vi "shooter_open.vi"(8 "error in (no error)":errorcluster) -> (0 "error out":errorcluster)   [LabVIEW 2020]
uses:
  <vilib>/Rock Robotics/WPI/ThirdParty/Phoenix-LabVIEW/Motor Controller/Controls/CTRE_Phoenix_MotorControl_NeutralMode.ctl
  Robot Global Data.vi
  <vilib>/Rock Robotics/WPI/ThirdParty/REV Robotics/REVLib/Typedef/Spark MAX Idle Mode.ctl
panel:
  in  "Turret PIDF Constants":T1={"Set Constants"=TRUE, "P"=0.02, "I"=0.0001, "D"=0.0, "F"=0.0, "I Zone"=0.0, "Cruise Velocity"=50000, "Acceleration"=50000, "Percent Deadband"=0.0}
  in  "Flywheel PIDF Constants":T1={"Set Constants"=TRUE, "P"=0.00029748, "I"=0.0, "D"=0.0, "F"=0.0, "I Zone"=0.0, "Cruise Velocity"=0, "Acceleration"=0, "Percent Deadband"=0.0}
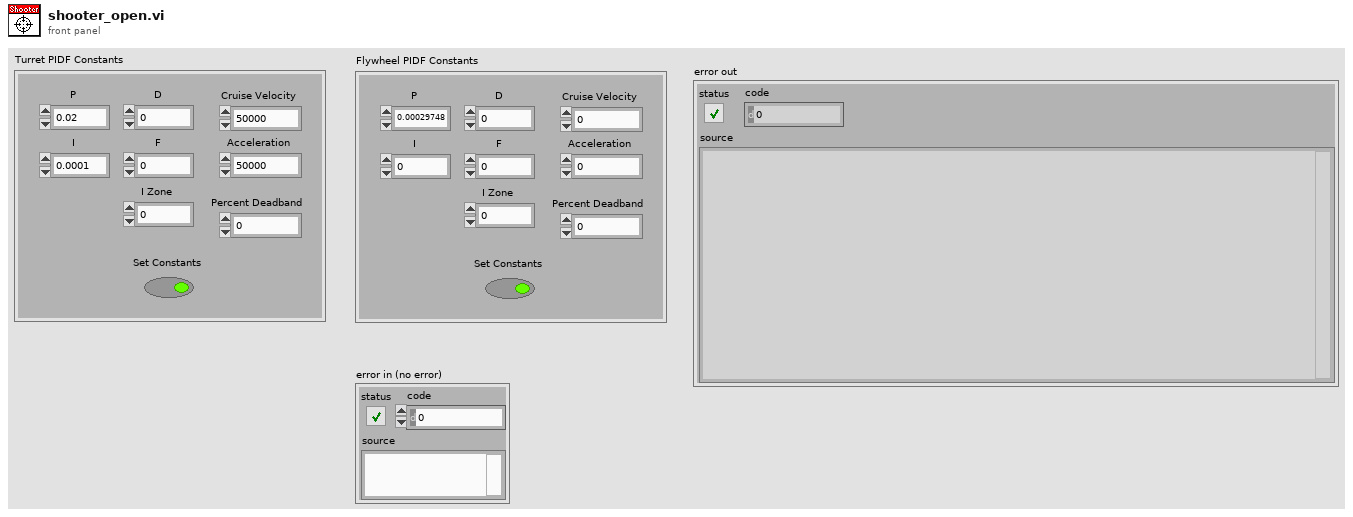
[diagram p1: front panel]
types:
  T1 = cluster{"Set Constants":bool, "P":dbl, "I":dbl, "D":dbl, "F":dbl, "I Zone":dbl, "Cruise Velocity":i32, "Acceleration":i32, "Percent Deadband":dbl}
  T2 = typedef "CTRE_Phoenix_MotorControl_NeutralMode.ctl" = enum8{"EEPROMSetting", "Override to Coast", "Override to Brake"}
  T3 = typedef "Spark MAX Idle Mode.ctl" = enum16{"Coast", "Brake"}
  T4 = typedef "WPI_MotorControlDeviceRef.ctl" = cluster{"DeviceStatus":errorcluster, "Type":T5, "PWM":cluster{"PWM Channel":T6, "DeadBand":T7}, "CAN":cluster{"Device Number":u8, "SetOutput VI Ref":variant, "GetOutput VI Ref":variant, "Enable VI Ref":variant, "Disable VI Ref":variant, "Data":variant}, "Invert":bool, "DIO PWM":cluster{"PWM \"Enable\" Channel":T6, "DIOChannel":T8, "PWM Rate":dbl}}
  T5 = typedef "WPI_MotorControlType.ctl" = enum16{"PWM", "CAN", "DIO PWM"}
  T6 = typedef "FPGA_DIOPWMChannel.ctl" = enum8{"PWM 0", "PWM 1", "PWM 2", "PWM 3", "PWM 4", "PWM 5", "PWM 6", "PWM 7", "PWM 8", "PWM 9", "PWM MXP 0", "PWM MXP 1", "PWM MXP 2", "PWM MXP 3", "PWM MXP 4", "PWM MXP 5", "PWM MXP 6", "PWM MXP 7", "PWM MXP 8", "PWM MXP 9", "Invalid"}
  T7 = typedef "WPI_PWMDeadband.ctl" = cluster{"Name":string, "maxPositivePwm":i32, "minPositivePwm":i32, "centerPwm":i32, "maxNegativePwm":i32, "minNegativePwm":i32, "angularRange":u16}
  T8 = typedef "FPGA_DIOChannel.ctl" = enum8{"DIO 0", "DIO 1", "DIO 2", "DIO 3", "DIO 4", "DIO 5", "DIO 6", "DIO 7", "DIO 8", "DIO 9", "DIO MXP 0", "DIO MXP 1", "DIO MXP 2", "DIO MXP 3", "DIO MXP 4", "DIO MXP 5", "DIO MXP 6", "DIO MXP 7", "DIO MXP 8", "DIO MXP 9", "DIO MXP 10", "DIO MXP 11", "DIO MXP 12", "DIO MXP 13", "DIO MXP 14", "DIO MXP 15", "SPI Port CS1", "SPI Port CS2", "SPI Port CS3", "SPI Port MISO", "SPI Port MOSI", "Invalid"}
  T9 = typedef "robot.ctl" = enum16{"Hyperion", "Theia"}
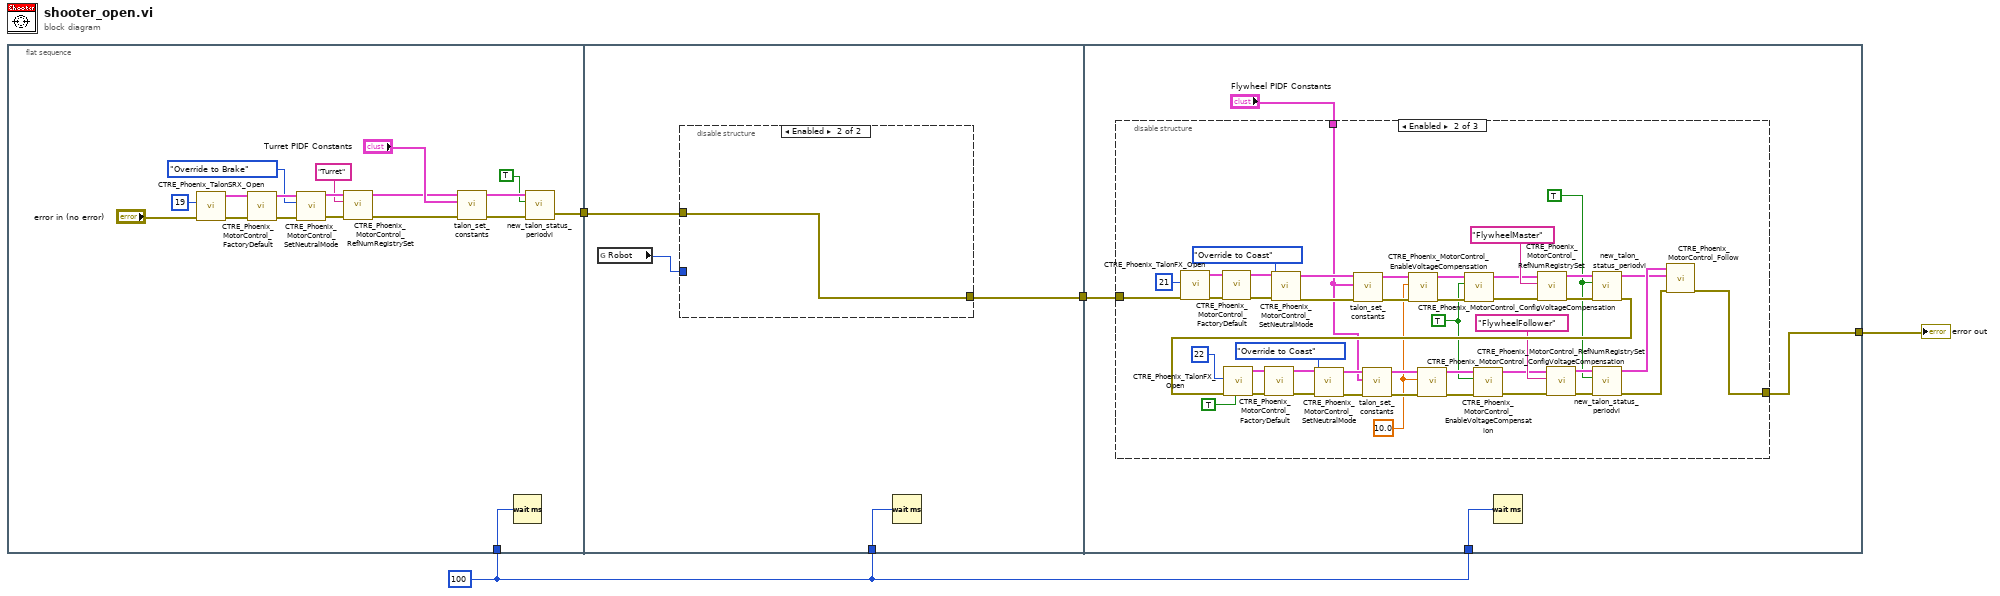
[diagram p0: block diagram]
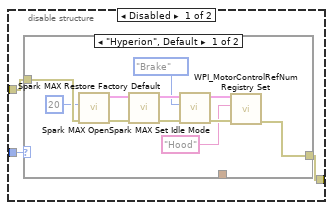
[diagram p2: hidden frame]
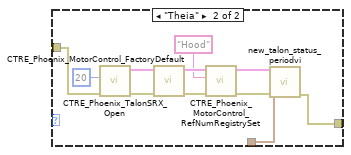
[diagram p3: hidden frame]
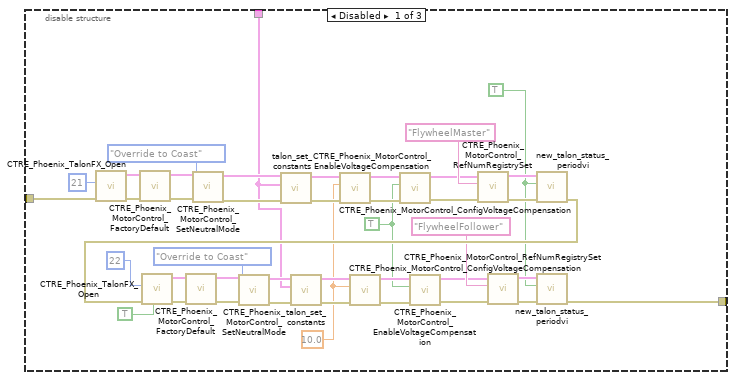
[diagram p4: hidden frame]
diagram:
  w1 = u32 100 ("milliseconds to wait")
  n1 = flat-sequence {
    tunnel: [w6] -> w4
    tunnel: w1 -> [w5]
    tunnel: w4 -> [w25]
    tunnel: [w24] -> w3
    tunnel: w1 -> [w23]
    tunnel: w3 -> [w56]
    tunnel: [w55] -> w2
    tunnel: w1 -> [w54]
    frame #0 {
      n2 = call <vilib>:"CTRE_Phoenix_TalonSRX_Open.vi"("error in"="error in (no error)", "Device Number"=u8 19) -> ("error out"=w17:errorcluster, "PhoenixMotorControlDevRef"=w16:T4)  [unwired: 8 in]
      n3 = call <vilib>:"CTRE_Phoenix_MotorControl_FactoryDefault.vi"("error in"=w17, "PhoenixMotorControlDevRef"=w16) -> ("error out"=w11:errorcluster, "PhoenixMotorControlDevRef"=w14:T4)  [unwired: 8 in]
      n4 = call <vilib>:"CTRE_Phoenix_MotorControl_SetNeutralMode.vi"("error in (no error)"=w11, "Motor Control Neutral Mode"=CTRE_Phoenix_MotorControl_NeutralMode."Override to Brake", "PhoenixMotorControlDevRef"=w14) -> ("error out"=w12:errorcluster, "PhoenixMotorControlDevRef"=w13:T4)  [unwired: 7 in]
      n5 = call <vilib>:"CTRE_Phoenix_MotorControl_RefNumRegistrySet.vi"("error in (no error)"=w12, "refnum name"="Turret", "PhoenixMotorControlDevRef"=w13) -> ("error out"=w19:errorcluster, "PhoenixMotorControlDevRef"=w18:T4)  [unwired: 7 in]
      n6 = call "talon_set_constants.vi"("error in"=w19, "Constants"="Turret PIDF Constants", "PhoenixMotorControlDevRef"=w18) -> ("error out"=w22:errorcluster, "PhoenixMotorControlDevRef"=w21:T4)  [unwired: 7 in]
      n7 = Wait (ms)(milliseconds to wait=w5) -> ()  [unwired: 1 out]
      n8 = call "new_talon_status_periodvi.vi"("error in (no error)"=w22, "Feedback Data?"=TRUE, "PhoenixMotorControlDevRef"=w21) -> ("error out"=w6:errorcluster)  [unwired: 7 in, 1 out]
    }
    frame #1 {
      n9 = global read "Robot Global Data.vi" "Robot"() -> (w26:T9)
      n10 = disable-structure shown="Enabled" {
        disable-tunnel: [w29 w52] -> w24
        disable-tunnel: w25 -> [w28 w52]
        disable-tunnel: w26 -> [w27 _]
        frame Disabled {
          n11 = case shown="\"Hyperion\", Default" w27 {
            tunnel: [w40 w41] -> w29
            tunnel: w28 -> [w39 w43]
            tunnel: _ -> [_ w42]
            frame "Hyperion", Default {
              n12 = call <vilib>:"Spark MAX Open.vi"("error in (no error)"=w39, "Device Number"=u8 20) -> ("error out"=w36:errorcluster, "MotorControlDeviceRef"=w37:T4)  [unwired: 8 in]
              n13 = call <vilib>:"Spark MAX Restore Factory Default.vi"("error in"=w36, "MotorControlDeviceRef"=w37) -> ("error out"=w35:errorcluster, "MotorControlDeviceRef"=w34:T4)  [unwired: 8 in]
              n14 = call <vilib>:"Spark MAX Set Idle Mode.vi"("error in (no error)"=w35, "Idle Mode"=Spark_MAX_Idle_Mode."Brake", "MotorControlDeviceRef in"=w34) -> ("error out"=w32:errorcluster, "MotorControlDeviceRef out"=w31:T4)  [unwired: 7 in]
              n15 = call <vilib>:"WPI_MotorControlRefNum Registry Set.vi"("error in (no error)"=w32, "refnum name"="Hood", "MotorControlDevRef"=w31) -> ("error out"=w40:errorcluster)  [unwired: 7 in, 1 out]
            }
            frame "Theia" {
              n16 = call <vilib>:"CTRE_Phoenix_TalonSRX_Open.vi"("error in"=w43, "Device Number"=u8 20) -> ("error out"=w46:errorcluster, "PhoenixMotorControlDevRef"=w47:T4)  [unwired: 8 in]
              n17 = call <vilib>:"CTRE_Phoenix_MotorControl_FactoryDefault.vi"("error in"=w46, "PhoenixMotorControlDevRef"=w47) -> ("error out"=w48:errorcluster, "PhoenixMotorControlDevRef"=w49:T4)  [unwired: 8 in]
              n18 = call <vilib>:"CTRE_Phoenix_MotorControl_RefNumRegistrySet.vi"("error in (no error)"=w48, "refnum name"="Hood", "PhoenixMotorControlDevRef"=w49) -> ("error out"=w51:errorcluster, "PhoenixMotorControlDevRef"=w50:T4)  [unwired: 7 in]
              n19 = call "new_talon_status_periodvi.vi"("error in (no error)"=w51, "Feedback Data?"=w42, "PhoenixMotorControlDevRef"=w50) -> ("error out"=w41:errorcluster)  [unwired: 7 in, 1 out]
            }
          }
        }
        frame Enabled {
        }
      }
      n20 = Wait (ms)(milliseconds to wait=w23) -> ()  [unwired: 1 out]
    }
    frame #2 {
      n21 = disable-structure shown="Enabled" {
        disable-tunnel: w56 -> [w74 w119 w144]
        disable-tunnel: [w73 w99 w144] -> w55
        disable-tunnel: "Flywheel PIDF Constants" -> [w57 w103 _]
        frame Disabled {
          w58 = TRUE ("Feedback Data?")
          w63 = TRUE ("Enable Voltage Compensation?")
          w64 = 10.0 ("Saturation Voltage")
          n22 = call <vilib>:"CTRE_Phoenix_TalonFX_Open.vi"("error in"=w74, "Device Number"=u8 21) -> ("error out"=w75:errorcluster, "PhoenixMotorControlDevRef"=w76:T4)  [unwired: 8 in]
          n23 = call <vilib>:"CTRE_Phoenix_MotorControl_FactoryDefault.vi"("error in"=w75, "PhoenixMotorControlDevRef"=w76) -> ("error out"=w80:errorcluster, "PhoenixMotorControlDevRef"=w79:T4)  [unwired: 8 in]
          n24 = call <vilib>:"CTRE_Phoenix_MotorControl_SetNeutralMode.vi"("error in (no error)"=w80, "Motor Control Neutral Mode"=CTRE_Phoenix_MotorControl_NeutralMode."Override to Coast", "PhoenixMotorControlDevRef"=w79) -> ("error out"=w96:errorcluster, "PhoenixMotorControlDevRef"=w95:T4)  [unwired: 7 in]
          n25 = call "talon_set_constants.vi"("error in"=w96, "Constants"=w57, "PhoenixMotorControlDevRef"=w95) -> ("error out"=w72:errorcluster, "PhoenixMotorControlDevRef"=w71:T4)  [unwired: 7 in]
          n26 = call <vilib>:"CTRE_Phoenix_MotorControl_ConfigVoltageCompensation.vi"("error in (no error)"=w72, "Saturation Voltage"=w64, "PhoenixMotorControlDevRef"=w71) -> ("error out"=w70:errorcluster, "PhoenixMotorControlDevRef"=w69:T4)  [unwired: 7 in]
          n27 = call <vilib>:"CTRE_Phoenix_MotorControl_EnableVoltageCompensation.vi"("error in (no error)"=w70, "Enable Voltage Compensation?"=w63, "PhoenixMotorControlDevRef"=w69) -> ("error out"=w61:errorcluster, "PhoenixMotorControlDevRef"=w62:T4)  [unwired: 7 in]
          n28 = call <vilib>:"CTRE_Phoenix_MotorControl_RefNumRegistrySet.vi"("error in (no error)"=w61, "refnum name"="FlywheelMaster", "PhoenixMotorControlDevRef"=w62) -> ("error out"=w92:errorcluster, "PhoenixMotorControlDevRef"=w94:T4)  [unwired: 7 in]
          n29 = call "new_talon_status_periodvi.vi"("error in (no error)"=w92, "Feedback Data?"=w58, "PhoenixMotorControlDevRef"=w94) -> ("error out"=w93:errorcluster)  [unwired: 7 in, 1 out]
          n30 = call <vilib>:"CTRE_Phoenix_TalonFX_Open.vi"("Invert"=TRUE, "error in"=w93, "Device Number"=u8 22) -> ("error out"=w82:errorcluster, "PhoenixMotorControlDevRef"=w83:T4)  [unwired: 7 in]
          n31 = call <vilib>:"CTRE_Phoenix_MotorControl_FactoryDefault.vi"("error in"=w82, "PhoenixMotorControlDevRef"=w83) -> ("error out"=w87:errorcluster, "PhoenixMotorControlDevRef"=w86:T4)  [unwired: 8 in]
          n32 = call <vilib>:"CTRE_Phoenix_MotorControl_SetNeutralMode.vi"("error in (no error)"=w87, "Motor Control Neutral Mode"=CTRE_Phoenix_MotorControl_NeutralMode."Override to Coast", "PhoenixMotorControlDevRef"=w86) -> ("error out"=w98:errorcluster, "PhoenixMotorControlDevRef"=w97:T4)  [unwired: 7 in]
          n33 = call "talon_set_constants.vi"("error in"=w98, "Constants"=w57, "PhoenixMotorControlDevRef"=w97) -> ("error out"=w66:errorcluster, "PhoenixMotorControlDevRef"=w65:T4)  [unwired: 7 in]
          n34 = call <vilib>:"CTRE_Phoenix_MotorControl_ConfigVoltageCompensation.vi"("error in (no error)"=w66, "Saturation Voltage"=w64, "PhoenixMotorControlDevRef"=w65) -> ("error out"=w67:errorcluster, "PhoenixMotorControlDevRef"=w68:T4)  [unwired: 7 in]
          n35 = call <vilib>:"CTRE_Phoenix_MotorControl_EnableVoltageCompensation.vi"("error in (no error)"=w67, "Enable Voltage Compensation?"=w63, "PhoenixMotorControlDevRef"=w68) -> ("error out"=w59:errorcluster, "PhoenixMotorControlDevRef"=w60:T4)  [unwired: 7 in]
          n36 = call <vilib>:"CTRE_Phoenix_MotorControl_RefNumRegistrySet.vi"("error in (no error)"=w59, "refnum name"="FlywheelFollower", "PhoenixMotorControlDevRef"=w60) -> ("error out"=w91:errorcluster, "PhoenixMotorControlDevRef"=w90:T4)  [unwired: 7 in]
          n37 = call "new_talon_status_periodvi.vi"("error in (no error)"=w91, "Feedback Data?"=w58, "PhoenixMotorControlDevRef"=w90) -> ("error out"=w73:errorcluster)  [unwired: 7 in, 1 out]
        }
        frame Enabled {
          w104 = TRUE ("Feedback Data?")
          w109 = TRUE ("Enable Voltage Compensation?")
          w110 = 10.0 ("Saturation Voltage")
          n38 = call <vilib>:"CTRE_Phoenix_TalonFX_Open.vi"("error in"=w119, "Device Number"=u8 21) -> ("error out"=w120:errorcluster, "PhoenixMotorControlDevRef"=w121:T4)  [unwired: 8 in]
          n39 = call <vilib>:"CTRE_Phoenix_MotorControl_FactoryDefault.vi"("error in"=w120, "PhoenixMotorControlDevRef"=w121) -> ("error out"=w125:errorcluster, "PhoenixMotorControlDevRef"=w124:T4)  [unwired: 8 in]
          n40 = call <vilib>:"CTRE_Phoenix_MotorControl_SetNeutralMode.vi"("error in (no error)"=w125, "Motor Control Neutral Mode"=CTRE_Phoenix_MotorControl_NeutralMode."Override to Coast", "PhoenixMotorControlDevRef"=w124) -> ("error out"=w141:errorcluster, "PhoenixMotorControlDevRef"=w140:T4)  [unwired: 7 in]
          n41 = call "talon_set_constants.vi"("error in"=w141, "Constants"=w103, "PhoenixMotorControlDevRef"=w140) -> ("error out"=w118:errorcluster, "PhoenixMotorControlDevRef"=w117:T4)  [unwired: 7 in]
          n42 = call <vilib>:"CTRE_Phoenix_MotorControl_ConfigVoltageCompensation.vi"("error in (no error)"=w118, "Saturation Voltage"=w110, "PhoenixMotorControlDevRef"=w117) -> ("error out"=w116:errorcluster, "PhoenixMotorControlDevRef"=w115:T4)  [unwired: 7 in]
          n43 = call <vilib>:"CTRE_Phoenix_MotorControl_EnableVoltageCompensation.vi"("error in (no error)"=w116, "Enable Voltage Compensation?"=w109, "PhoenixMotorControlDevRef"=w115) -> ("error out"=w107:errorcluster, "PhoenixMotorControlDevRef"=w108:T4)  [unwired: 7 in]
          n44 = call <vilib>:"CTRE_Phoenix_MotorControl_RefNumRegistrySet.vi"("error in (no error)"=w107, "refnum name"="FlywheelMaster", "PhoenixMotorControlDevRef"=w108) -> ("error out"=w137:errorcluster, "PhoenixMotorControlDevRef"=w139:T4)  [unwired: 7 in]
          n45 = call "new_talon_status_periodvi.vi"("error in (no error)"=w137, "Feedback Data?"=w104, "PhoenixMotorControlDevRef"=w139) -> ("error out"=w138:errorcluster, "PhoenixMotorControlDevRef"=w100:T4)  [unwired: 7 in]
          n46 = call <vilib>:"CTRE_Phoenix_TalonFX_Open.vi"("Invert"=TRUE, "error in"=w138, "Device Number"=u8 22) -> ("error out"=w127:errorcluster, "PhoenixMotorControlDevRef"=w128:T4)  [unwired: 7 in]
          n47 = call <vilib>:"CTRE_Phoenix_MotorControl_FactoryDefault.vi"("error in"=w127, "PhoenixMotorControlDevRef"=w128) -> ("error out"=w132:errorcluster, "PhoenixMotorControlDevRef"=w131:T4)  [unwired: 8 in]
          n48 = call <vilib>:"CTRE_Phoenix_MotorControl_SetNeutralMode.vi"("error in (no error)"=w132, "Motor Control Neutral Mode"=CTRE_Phoenix_MotorControl_NeutralMode."Override to Coast", "PhoenixMotorControlDevRef"=w131) -> ("error out"=w143:errorcluster, "PhoenixMotorControlDevRef"=w142:T4)  [unwired: 7 in]
          n49 = call "talon_set_constants.vi"("error in"=w143, "Constants"=w103, "PhoenixMotorControlDevRef"=w142) -> ("error out"=w112:errorcluster, "PhoenixMotorControlDevRef"=w111:T4)  [unwired: 7 in]
          n50 = call <vilib>:"CTRE_Phoenix_MotorControl_ConfigVoltageCompensation.vi"("error in (no error)"=w112, "Saturation Voltage"=w110, "PhoenixMotorControlDevRef"=w111) -> ("error out"=w113:errorcluster, "PhoenixMotorControlDevRef"=w114:T4)  [unwired: 7 in]
          n51 = call <vilib>:"CTRE_Phoenix_MotorControl_EnableVoltageCompensation.vi"("error in (no error)"=w113, "Enable Voltage Compensation?"=w109, "PhoenixMotorControlDevRef"=w114) -> ("error out"=w105:errorcluster, "PhoenixMotorControlDevRef"=w106:T4)  [unwired: 7 in]
          n52 = call <vilib>:"CTRE_Phoenix_MotorControl_RefNumRegistrySet.vi"("error in (no error)"=w105, "refnum name"="FlywheelFollower", "PhoenixMotorControlDevRef"=w106) -> ("error out"=w136:errorcluster, "PhoenixMotorControlDevRef"=w135:T4)  [unwired: 7 in]
          n53 = call "new_talon_status_periodvi.vi"("error in (no error)"=w136, "Feedback Data?"=w104, "PhoenixMotorControlDevRef"=w135) -> ("error out"=w101:errorcluster, "PhoenixMotorControlDevRef"=w102:T4)  [unwired: 7 in]
          n54 = call <vilib>:"CTRE_Phoenix_MotorControl_Follow.vi"("error in (no error)"=w101, "Master Controller to Follow"=w100, "PhoenixMotorControlDevRef"=w102) -> ("error out"=w99:errorcluster)  [unwired: 7 in, 1 out]
        }
        frame Disabled {
        }
      }
      n55 = Wait (ms)(milliseconds to wait=w54) -> ()  [unwired: 1 out]
    }
  }
  "error out" <- w2
